vi "header.vi"(8 "errorIn":errorcluster, 11 "xmlRef":refnum<k20>) -> (0 "errorOut":errorcluster, 2 "header":T1, 3 "xmlRef":refnum<k20>)   [LabVIEW 2017]
uses:
  models/Header.ctl
  <vilib>/xml/Close Reference(Node).vi
  <vilib>/xml/Close Reference(NdList).vi
  <resource>/objmgr/DOMUserDefRef.rc
  <vilib>/xml/NI_XML.lvlib
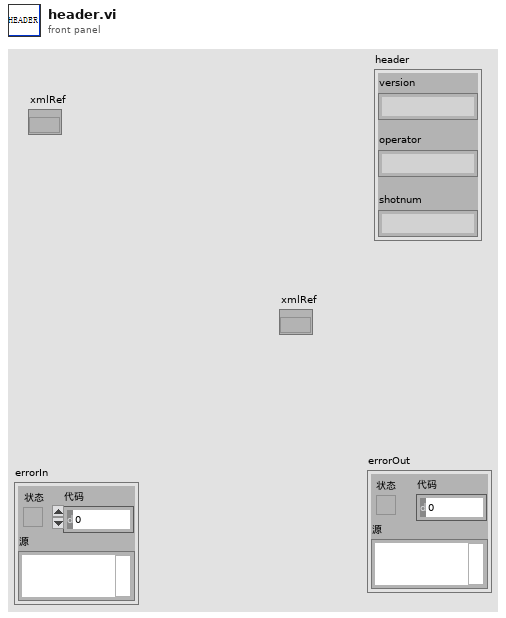
[diagram p1: front panel]
types:
  T1 = typedef "Header.ctl" = cluster{"version":string, "operator":string, "shotnum":string}
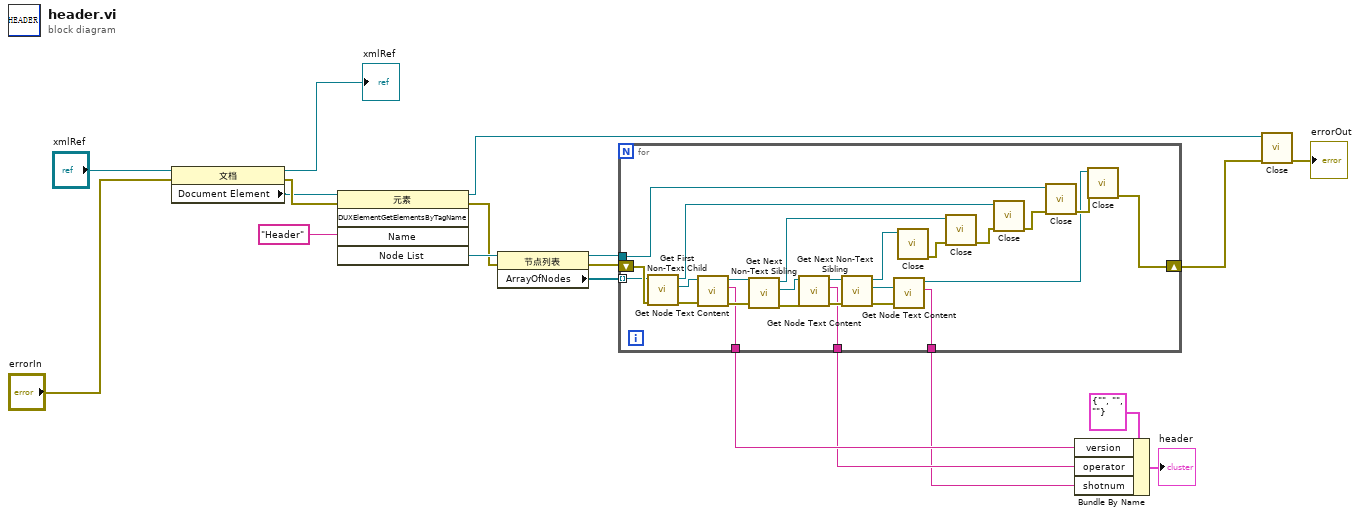
[diagram p0: block diagram]
diagram:
  n1 = property class="文档"(reference="xmlRef", error in="errorIn") -> (reference out=→"xmlRef":refnum<k20>, error out=w14:errorcluster, "Document Element"=w9:refnum<k20>)
  n2 = invoke class="元素" method="DUXElementGetElementsByTagName"(reference=w9, error in=w14, "Name"="Header" ("Node Name")) -> (reference out=w13:refnum<k20>, error out=w17:errorcluster, "Node List"=w18:refnum<k20>)  [unwired: 2 in, 2 out]
  n3 = property class="节点列表"(reference=w18, error in=w17) -> (reference out=w16:refnum<k20>, error out=w15:errorcluster, "ArrayOfNodes"=w12:refnum<k20>[])
  n4 = for {
    tunnel: w12 -> [w26] mode=indexing
    tunnel: w16 -> [w29]
    shift-right: [w23] -> w10
    shift-left: w15 -> [w28]
    tunnel: [w22] -> w4
    tunnel: [w21] -> w3
    tunnel: [w20] -> w2
    n5 = call <vilib>:"Get First Non-Text Child.vi"("error in (no error)"=w28, "node in"=w26) -> ("error out"=w43:errorcluster, "child node"=w44:refnum<k20>, "node out"=w36:refnum<k20>)  [unwired: 7 out]
    n6 = call <vilib>:"Get Node Text Content.vi"("error in (no error)"=w43, "node in"=w44) -> ("error out"=w39:errorcluster, "node text"=w22:string, "node out"=w40:refnum<k20>)  [unwired: 7 out]
    n7 = call <vilib>:"Get Next Non-Text Sibling.vi"("error in (no error)"=w39, "node in"=w40) -> ("error out"=w42:errorcluster, "sibling node"=w41:refnum<k20>, "node out"=w38:refnum<k20>)  [unwired: 7 out]
    n8 = call <vilib>:"Get Node Text Content.vi"("error in (no error)"=w42, "node in"=w41) -> ("error out"=w32:errorcluster, "node text"=w21:string, "node out"=w34:refnum<k20>)  [unwired: 7 out]
    n9 = call <vilib>:"Get Next Non-Text Sibling.vi"("error in (no error)"=w32, "node in"=w34) -> ("error out"=w31:errorcluster, "sibling node"=w30:refnum<k20>, "node out"=w33:refnum<k20>)  [unwired: 7 out]
    n10 = call <vilib>:"Get Node Text Content.vi"("error in (no error)"=w31, "node in"=w30) -> ("node text"=w20:string, "node out"=w24:refnum<k20>)  [unwired: 8 out]
    n11 = call-poly <vilib>:"Close.vi"("node"=w33) -> ("error out"=w37:errorcluster)  [unwired: 1 in, 7 out]
    n12 = call-poly <vilib>:"Close.vi"("error in (no error)"=w37, "node"=w38) -> ("error out"=w35:errorcluster)  [unwired: 7 out]
    n13 = call-poly <vilib>:"Close.vi"("error in (no error)"=w35, "node"=w36) -> ("error out"=w27:errorcluster)  [unwired: 7 out]
    n14 = call-poly <vilib>:"Close.vi"("error in (no error)"=w27, "node list"=w29) -> ("error out"=w25:errorcluster)  [unwired: 7 out]
    n15 = call-poly <vilib>:"Close.vi"("error in (no error)"=w25, "node"=w24) -> ("error out"=w23:errorcluster)  [unwired: 7 out]
  }
  n16 = Bundle By Name(cluster=T1 {"version"="", "operator"="", "shotnum"=""} ("Header"), "version"=w4, "operator"=w3, "shotnum"=w2) -> (→"header":T1)
  n17 = call-poly <vilib>:"Close.vi"("error in (no error)"=w10, "node"=w13) -> ("error out"=→"errorOut":errorcluster)  [unwired: 7 out]
